vi "Switch Box Auto Mode Control.vi"(0 "PhyChls":tag="Dev1/port0/line4", 1 "line grouping":i32(ring) items=["one channel for each line", "one channel for all lines"], 5 "OFF/ON":bool, 7 "Invert":bool, 11 "ErrIn":errorcluster, 12 "SimOn":bool, 13 "Init":bool, 14 "Stop":bool) -> (15 "ErrOut":errorcluster)   [LabVIEW 2013]
uses:
  <vilib>/DAQmx/write.llb/DAQmx Write (Digital Bool 1Line 1Point).vi
  <vilib>/DAQmx/create/channels.llb/DAQmx Create Channel (DO-Digital Output).vi
  <vilib>/DAQmx/miscellaneous.llb/DAQmx Fill In Error Info.vi
panel:
  # "ER2007"
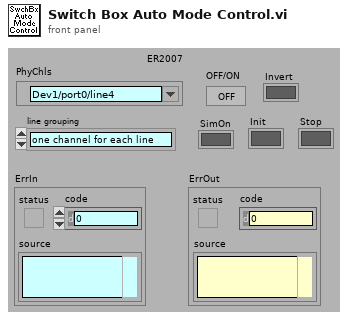
[diagram p1: front panel]
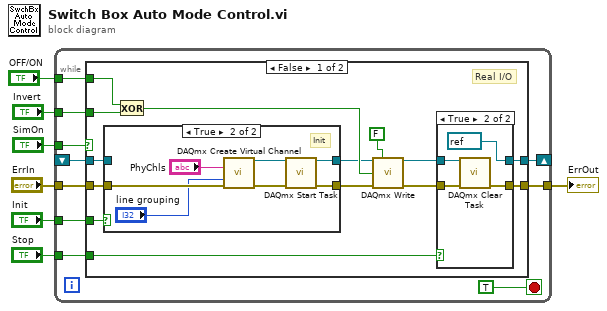
[diagram p0: block diagram]
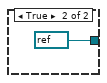
[diagram p5: hidden frame]
diagram:
  n1 = while {
    tunnel: "ErrIn" -> [w17]
    tunnel: [w16] -> w6
    tunnel: "SimOn" -> [w15]
    tunnel: "Stop" -> [w14]
    tunnel: "Init" -> [w13]
    shift-right: [w11] -> _
    shift-left: _ -> [w10]
    tunnel: "Invert" -> [w9]
    tunnel: "OFF/ON" -> [w8]
    stop <- TRUE stop-if-true
    n2 = case shown="False" w15 {
      tunnel: w17 -> [w31 w50]
      tunnel: [w29 w50] -> w16
      tunnel: w14 -> [w30 _]
      tunnel: w13 -> [w22 w49]
      tunnel: [w21 w48] -> w11
      tunnel: w10 -> [w20 w47]
      tunnel: w9 -> [w19 _]
      tunnel: w8 -> [w18 _]
      frame False {
        # "Real I/O"
        n3 = case shown="True" w22 {
          tunnel: w31 -> [w32 w40]
          tunnel: [w32 w36] -> w24
          tunnel: [w33 w34] -> w23
          tunnel: w20 -> [w33 _]
          frame False {
          }
          frame True {
            # "Init"
            n4 = call-poly <vilib>:"DAQmx Create Virtual Channel.vi"("lines"="PhyChls", "line grouping"="line grouping", "error in"=w40) -> ("task out"=w35:refnum<k21>, "error out"=w37:errorcluster)  [unwired: 11 in]
            n5 = call <vilib>:"DAQmx Start Task.vi"("task/channels in"=w35, "error in"=w37) -> ("task out"=w34:refnum<k21>, "error out"=w36:errorcluster)  [unwired: 12 in]
          }
        }
        n6 = Exclusive Or(1:w19, 2:w18) -> (0:w27:bool)
        n7 = call-poly <vilib>:"DAQmx Write.vi"("task/channels in"=w23, "auto start"=FALSE, "data"=w27, "error in"=w24) -> ("task out"=w25:refnum<k21>, "error out"=w26:errorcluster)  [unwired: 9 in, 1 out]
        n8 = case shown="True" w30 {
          tunnel: w26 -> [w42 w46]
          tunnel: w25 -> [w41 w45]
          tunnel: [w42 w44] -> w29
          tunnel: [w41 refnum<k21> refnum ("task out")] -> w21
          frame False {
          }
          frame True {
            n9 = call <vilib>:"DAQmx Clear Task.vi"("task in"=w45, "error in"=w46) -> ("error out"=w44:errorcluster)  [unwired: 13 in]
          }
        }
      }
      frame True {
        # "Simulation"
        n10 = case shown="False" w49 {
          tunnel: [w51 refnum<k21> refnum ("task out")] -> w48
          tunnel: w47 -> [w51 _]
          frame False {
          }
          frame True {
          }
        }
      }
    }
  }
  "ErrOut" <- w6
